vi "oa_Check Continuity of Even Angle Signal.vi"(8 "averaging revolution (1)":dbl=1.0 min=0.0, 9 "averaging type":enum16{"Linear (default)", "Exponential", "Mix"}(ring), 10 "even angle signal":cluster{"r0":dbl, "dr":dbl, "Y":dbl[]}={"r0"=0.0, "dr"=1.0, "Y"=[]} {"r0" format="%.2p"; "dr" format="%.2p"; "Y" format="%.2f"}, 11 "reset?(F)":bool) -> (0 "dul averaging revolution":dbl, 1 "dul averaging type":enum16{"Linear (default)", "Exponential", "Mix"}(ring), 2 "dul even angle signal":cluster{"r0":dbl, "dr":dbl, "Y":dbl[]}={"r0"=0.0, "dr"=1.0, "Y"=[]} {"r0" format="%.2p"; "dr" format="%.2p"; "Y" format="%.2f"}, 3 "reset out":bool, 4 "points/rev":u32)   [LabVIEW 2017, in "SoundVib_OAUtility.lvlib"]
uses:
  <vilib>/addons/Sound and Vibration/Order Analysis/Utility/SoundVib_OAUtility.lvlib
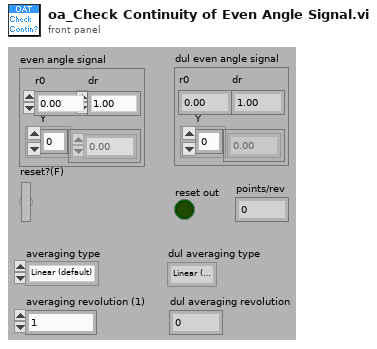
[diagram p1: front panel]
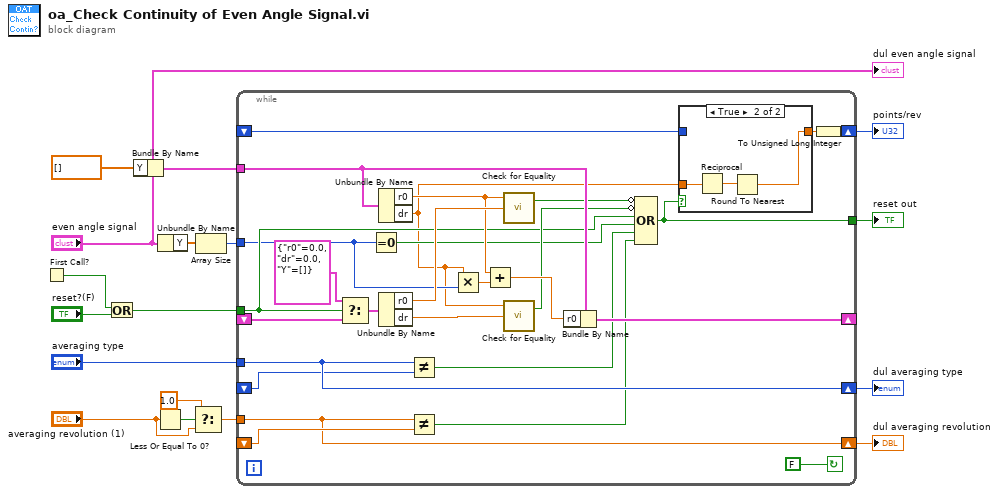
[diagram p0: block diagram]
diagram:
  n1 = First Call?() -> (First Call?: T/F=w13:bool)
  n2 = Or(x=w13, y="reset?(F)") -> (x .or. y?=w11:bool)
  n3 = Bundle By Name(cluster="even angle signal", "Y"=dbl[] []) -> (w17:cluster{"r0":dbl, "dr":dbl, "Y":dbl[]})
  n4 = Less Or Equal To 0?(x="averaging revolution (1)") -> (x <= 0?=w4:bool)
  n5 = Unbundle By Name("even angle signal") -> ("Y"=w9:dbl[])
  n6 = Select(t=1.0, s=w4, f="averaging revolution (1)") -> (s? t:f=w3:dbl)
  n7 = Array Size(array=w9) -> (size(s)=w15:i32)
  n8 = while {
    shift-right: [w41] -> _
    shift-left: _ -> [w34]
    tunnel: w17 -> [w42]
    tunnel: w15 -> [w30]
    tunnel: [w25] -> w12
    tunnel: w11 -> [w31]
    tunnel: "averaging type" -> [w28]
    shift-right: [w28] -> w6
    shift-left: _ -> [w27]
    shift-right: [w22] -> w8
    shift-left: _ -> [w23]
    shift-right: [w19] -> w5
    shift-left: _ -> [w20]
    tunnel: w3 -> [w19]
    stop <- FALSE continue-if-true
    n9 = Select(t=cluster{"r0":dbl, "dr":dbl, "Y":dbl[]} {"r0"=0.0, "dr"=0.0, "Y"=[]} ("even angle signal"), s=w31, f=w34) -> (s? t:f=w33:cluster{"r0":dbl, "dr":dbl, "Y":dbl[]})
    n10 = Equal To 0?(x=w30) -> (x = 0?=w29:bool)
    n11 = Unbundle By Name(w42) -> ("r0"=w37:dbl, "dr"=w24:dbl)
    n12 = Unbundle By Name(w33) -> ("r0"=w39:dbl, "dr"=w43:dbl)
    n13 = Not Equal?(x=w28, y=w27) -> (x != y?=w26:bool)
    n14 = Not Equal?(x=w19, y=w20) -> (x != y?=w18:bool)
    n15 = Multiply(x=w24, y=w30) -> (x*y=w40:dbl)
    n16 = Add(x=w37, y=w40) -> (x+y=w38:dbl)
    n17 = call <vilib>:"Check for Equality.vi"("n2"=w39, "n1"=w37) -> ("equal?"=w36:bool)  [unwired: 1 in, 1 out]
    n18 = call <vilib>:"Check for Equality.vi"("n2"=w43, "n1"=w24) -> ("equal?"=w35:bool)  [unwired: 1 in, 1 out]
    n19 = Bundle By Name(cluster=w42, "r0"=w38) -> (w41:cluster{"r0":dbl, "dr":dbl, "Y":dbl[]})
    n20 = Compound Arithmetic op=OR(invert w36, invert w35, w31, w29, w26, w18) -> (w25:bool)
    n21 = case shown="True" w25 {
      tunnel: w24 -> [_ w48]
      tunnel: [w45 w46] -> w21
      tunnel: w23 -> [w45 _]
      frame False {
      }
      frame True {
        n22 = Reciprocal(x=w48) -> (1/x=w47:dbl)
        n23 = Round To Nearest(number=w47) -> (nearest integer value=w46:dbl)
      }
    }
    n24 = To Unsigned Long Integer(number=w21) -> (unsigned 32bit integer=w22:u32)
  }
  "reset out" <- w12
  "points/rev" <- w8
  "dul averaging type" <- w6
  "dul averaging revolution" <- w5
  "dul even angle signal" <- "even angle signal"
